vi "选择模块.vi"() -> ()   [LabVIEW 2016]
uses:
  <vilib>/Utility/sysdir.llb/System Directory Type.ctl
panel:
  out "名称或相对路径":string
  in  "枚举":enum16{"模块一", "模块二"}(ring)
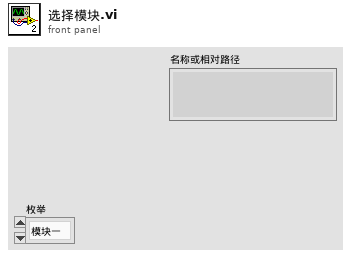
[diagram p1: front panel]
types:
  T1 = typedef "System Directory Type.ctl" = i32
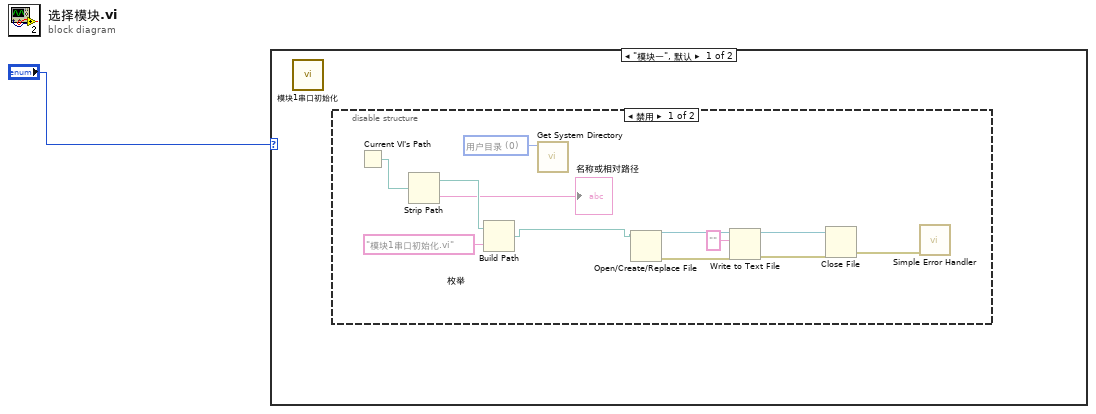
[diagram p0: block diagram]
diagram:
  n1 = case shown="\"模块一\", 默认" "枚举" {
    frame "模块一", Default {
      n2 = call "模块1串口初始化.vi"() -> ()  [unwired: 12 in]
      n3 = disable-structure shown="禁用" {
        frame Disabled {
          w9 = T1 0 items=["用户目录"=0, "用户桌面"=1, "用户文档"=2, "用户应用程序数据"=3, "用户设置"=4, "用户临时目录"=5, "公共文档"=6, "公共应用程序数据"=7, "公共设置"=8, "公共缓存"=13, "系统核心库"=9, "系统安装库"=10, "应用程序文件"=11, "启动盘根目录"=12] ("system directory type")
          n4 = Current VI's Path() -> (path=w8:path)
          n5 = Strip Path(path=w8) -> (stripped path=w11:path, name=→"名称或相对路径":string)
          n6 = Build Path(base path=w11, name or relative path="模块1串口初始化.vi" ("名称或相对路径")) -> (appended path=w13:path)
          n7 = call <vilib>:"Get System Directory.vi"("system directory type"=w9) -> ()  [unwired: 10 in, 1 out]
          n8 = Open/Create/Replace File(file path (use dialog)=w13) -> (refnum out=w7:refnum<file>, error out=w5:errorcluster)  [unwired: 5 in, 1 out]
          n9 = Write to Text File(file (use dialog)=w7, text="" ("文本"), error in=w5) -> (refnum out=w6:refnum<file>, error out=w4:errorcluster)  [unwired: 1 in, 1 out]
          n10 = Close File(refnum=w6, error in=w4) -> (error out=w3:errorcluster)  [unwired: 1 out]
          n11 = call <vilib>:"Simple Error Handler.vi"("error in (no error)"=w3) -> ()  [unwired: 4 in, 5 out]
        }
        frame Enabled {
        }
      }
    }
    frame "模块二" {
    }
  }
